vi "Regex Match.vi"(10 "regular expression":string, 11 "string":string) -> (3 "match?":bool)   [LabVIEW 2018, in "Utilities.lvlib"]
uses:
  Utilities.lvlib
  <vilib>/regexp/Match Regular Expression.xnode
panel:
  # "Connector Pane"
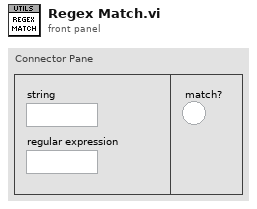
[diagram p1: front panel]
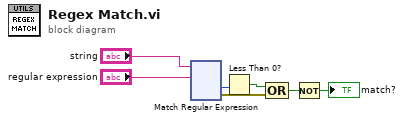
[diagram p0: block diagram]
diagram:
  n1 = xnode "Match Regular Expression"("input string"="string", "regular expression"="regular expression") -> ("offset past match"=w5:i32, "error out"=w1:errorcluster)  [unwired: 4 in, 3 out]
  n2 = Less Than 0?(x=w5) -> (x < 0?=w6:bool)
  n3 = Compound Arithmetic op=OR(w6, w1) -> (w7:bool)
  n4 = Not(x=w7) -> (.not. x?=→"match?":bool)
